vi "Interface_Asset_Get Parameter Control Refs.vi"(8 "error in (no error)":errorcluster, 11 "EnergyStorage in":refnum<class "EnergyStorage.lvclass">) -> (0 "error out":errorcluster, 2 "Controls[]":refnum<vi>[](array[refnum]), 3 "EnergyStorage out":refnum<class "EnergyStorage.lvclass">)   [LabVIEW 2015, in "EnergyStorage.lvclass"]
uses:
  EnergyStorage.lvclass
  EnergyStorage_Status.ctl
  EnergyStorage_Control.ctl
  EnergyStorage.lvclass/EnergyStorage.ctl
panel:
  out "Control":T1
  out "Status":T2
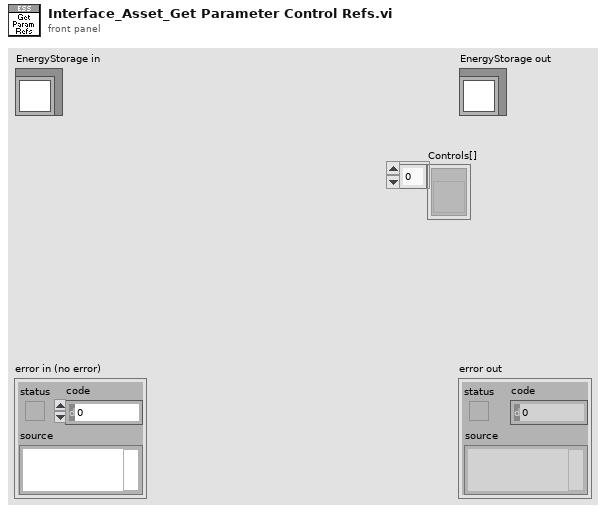
[diagram p1: front panel]
types:
  T1 = typedef "EnergyStorage.lvclass/EnergyStorage_Control.ctl" = cluster{"kW Setpoint":dbl}
  T2 = typedef "EnergyStorage.lvclass/EnergyStorage_Status.ctl" = cluster{"kW":dbl, "SOC":dbl}
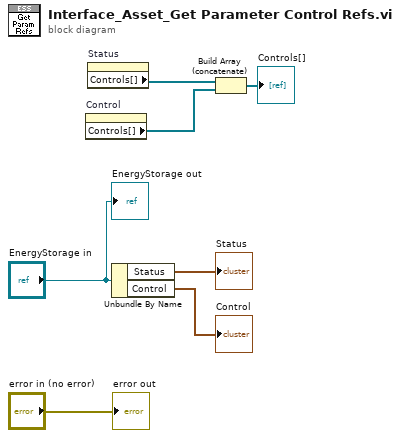
[diagram p0: block diagram]
diagram:
  n1 = property on="Control" class="Clust (strict)"() -> ("Controls[]"=w3:refnum<vi>[])  [unwired: 2 in, 2 out]
  n2 = property on="Status" class="Clust (strict)"() -> ("Controls[]"=w2:refnum<vi>[])  [unwired: 2 in, 2 out]
  n3 = Unbundle By Name("EnergyStorage in") -> ("Status"=→"Status":T2, "Control"=→"Control":T1)
  n4 = Build Array (concatenate)(w2, w3) -> (→"Controls[]":refnum<vi>[])
  "error out" <- "error in (no error)"
  "EnergyStorage out" <- "EnergyStorage in"
